vi "MAIN_start_acquiring.vi"(4 "error in":errorcluster, 5 "queue MAIN":refnum<queue>, 6 "Image contrast":cluster{i32, i32}(slide)={16000, 0} scale=0.0..16000.0, 7 "queue CAMERA":refnum<queue>) -> (0 "error out":errorcluster)   [LabVIEW 2015]
uses:
  CONTROLS/Q_main_element.ctl
  CONTROLS/Q_camera_element.ctl
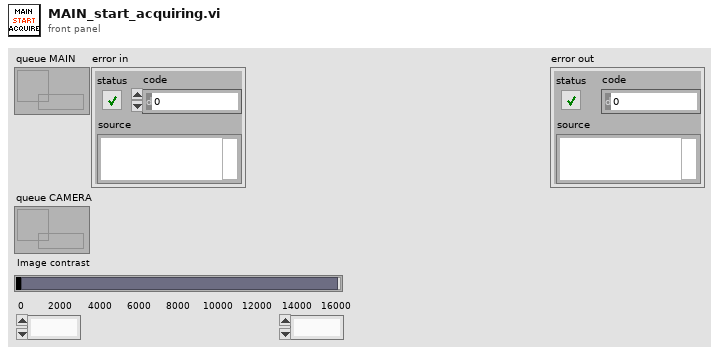
[diagram p1: front panel]
types:
  T1 = typedef "Q_camera_element.ctl" = cluster{"variant":variant, "Instruction":enum16{"CAMERA_idle", "CAMERA_initialize", "CAMERA_error", "CAMERA_security_stop", "CAMERA_not_acquiring", "CAMERA_acquiring", "CAMERA_start_acquiring", "CAMERA_stop_acquiring", "CAMERA_change_exposure", "CAMERA_define_ROI", "CAMERA_cooler", "CAMERA_acquire_movie", "CAMERA_init_scan", "CAMERA_check_image_scan", "CAMERA_close_scan", "CAMERA_init_merFISH", "CAMERA_start_acquiring_merFISH", "CAMERA_close_scan_merFISH", "CAMERA_close_merFISH", "CAMERA_STOP"}}
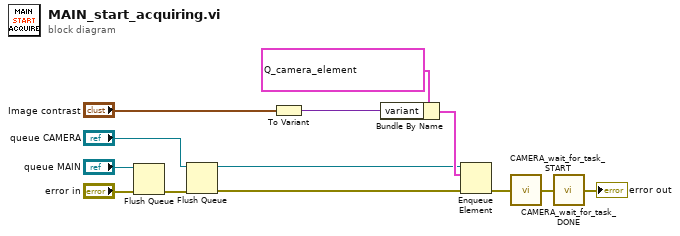
[diagram p0: block diagram]
diagram:
  n1 = Flush Queue(queue="queue MAIN", error in (no error)="error in") -> (error out=w9:errorcluster)  [unwired: 2 out]
  n2 = Flush Queue(queue="queue CAMERA", error in (no error)=w9) -> (queue out=w8:refnum<queue>, error out=w7:errorcluster)  [unwired: 1 out]
  n3 = To Variant(anything="Image contrast") -> (Variant=w10:variant)
  n4 = Bundle By Name(cluster=T1 {"variant"=variant, "Instruction"=enum."CAMERA_start_acquiring"} ("Q_ANDOR_element"), "variant"=w10) -> (w11:T1)
  n5 = Enqueue Element(queue=w8, element=w11, error in (no error)=w7) -> (error out=w2:errorcluster)  [unwired: 1 in, 2 out]
  n6 = call "CAMERA_wait_for_task_START.vi"("error in"=w2) -> ("error out"=w12:errorcluster)
  n7 = call "CAMERA_wait_for_task_DONE.vi"("error in"=w12) -> ("error out"=→"error out":errorcluster)
